vi "String to mission Select.vi"(8 "error in":errorcluster, 11 "Test Selector in":refnum<class "Test Selector.lvclass">) -> (0 "error out":errorcluster, 1 "Test Dialog":string, 3 "Test Selector out":refnum<class "Test Selector.lvclass">)   [LabVIEW 2019, in "Test Selector.lvlib" / "Test Selector.lvclass"]
uses:
  Test Selector.lvclass
  Test Selector.lvclass/Test Selector.ctl
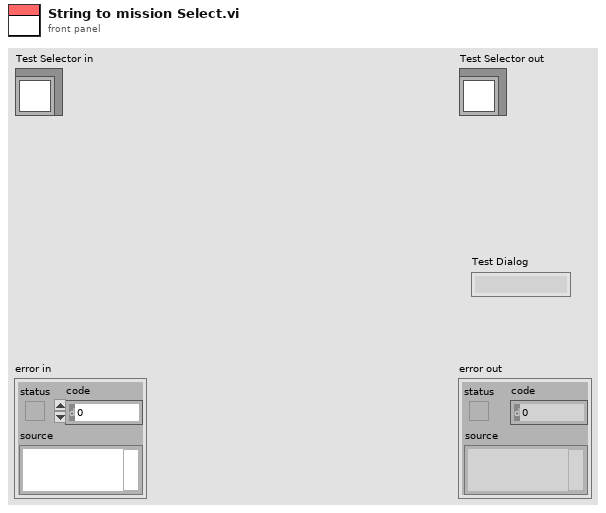
[diagram p1: front panel]
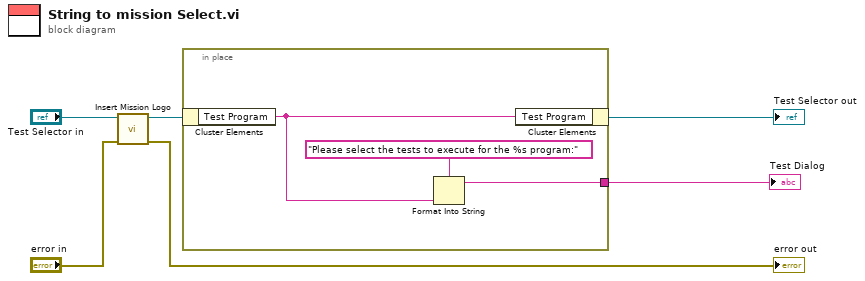
[diagram p0: block diagram]
diagram:
  n1 = call "Insert Mission Logo.vi"("error in"="error in", "Test Selector in"="Test Selector in") -> ("error out"=→"error out":errorcluster, "Test Selector out"=w2:refnum<class "Test Selector.lvclass">)  [unwired: 8 in]
  n2 = in-place {
    in-place-border: [w7] -> w5
    n3 = in-place-cluster #1(w2) -> ("Test Program"=w9:string)
    n4 = Format Into String(format string="Please select the tests to execute for the %s program:", w9) -> (resulting string=w7:string)  [unwired: 2 in, 1 out]
    n5 = in-place-cluster #1("Test Program"=w9) -> (→"Test Selector out":refnum<class "Test Selector.lvclass">)
  }
  "Test Dialog" <- w5
